vi "Write gRPCid.vi"(8 "error in (no error)":errorcluster, 10 "gRPCid":T1, 11 "MeasurementPluginService in":refnum<class "Measurement Plugin Service.lvclass">) -> (0 "error out":errorcluster, 3 "MeasurementPluginService out":refnum<class "Measurement Plugin Service.lvclass">)   [LabVIEW 2020, in "MeasurementLink Measurement Server.lvlib" / "Measurement Plugin Service.lvclass"]
uses:
  Measurement Plugin Service.lvclass
  <vilib>/gRPC/LabVIEW gRPC Library/Shared/grpcId.ctl
  <vilib>/gRPC/LabVIEW gRPC Library/grpc-lvsupport-release.lvlib
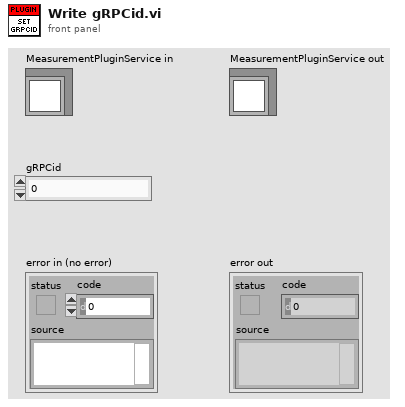
[diagram p1: front panel]
types:
  T1 = typedef "grpc-lvsupport-release.lvlib/grpcId.ctl" = u64
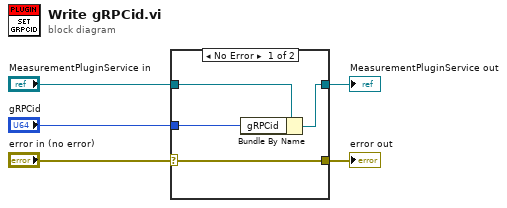
[diagram p0: block diagram]
diagram:
  n1 = case shown="No Error" "error in (no error)" {
    selector: "error in (no error)" -> [w9 w10]
    tunnel: [w9 w10] -> w4
    tunnel: [w7 w11] -> w2
    tunnel: "MeasurementPluginService in" -> [w8 w11]
    tunnel: "gRPCid" -> [w6 _]
    frame No Error {
      n2 = Bundle By Name(cluster=w8, "gRPCid"=w6) -> (w7:refnum<class "Measurement Plugin Service.lvclass">)
    }
    frame Error {
    }
  }
  "error out" <- w4
  "MeasurementPluginService out" <- w2
